vi "Volts_to_temperature_PT__(SubVI).vi"(1 "делитель":dbl, 4 "Resistance":i32, 7 "error in":errorcluster, 16 "Cluster":cluster{"Rref":ext, "Tref":ext, "k":ext}) -> (9 "s? color":u32, 10 "Vin < 0?":bool, 20 "T solvation":dbl, 21 "meas_voltage":dbl, 27 "error out":errorcluster)   [LabVIEW 2015]
uses:
  <vilib>/express/express arith-compare/Formula/XNode/ExpressFormulaBlockNode.xnode
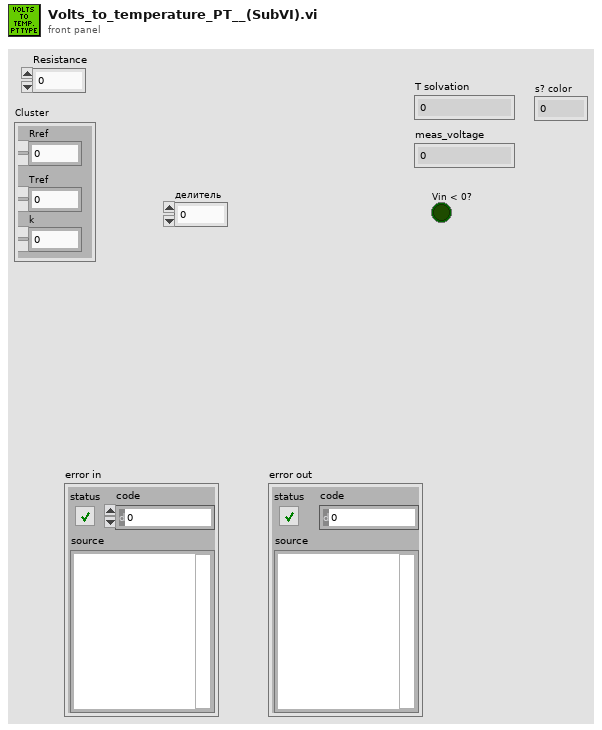
[diagram p1: front panel]
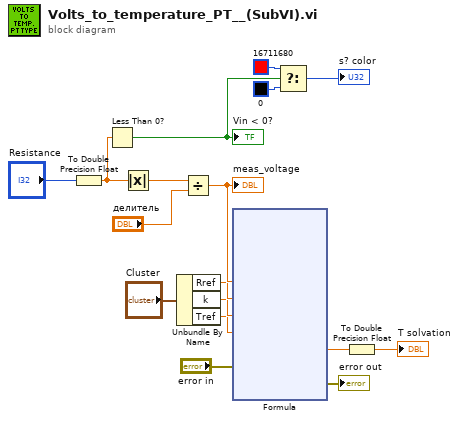
[diagram p0: block diagram]
diagram:
  n1 = To Double Precision Float(number="Resistance") -> (double precision float=w1:dbl)
  n2 = Less Than 0?(x=w1) -> (x < 0?=w15:bool)
  "Vin < 0?" <- w15
  n3 = Absolute Value(x=w1) -> (abs(x)=w13:dbl)
  n4 = Unbundle By Name("Cluster") -> ("Rref"=w5:ext, "k"=w4:ext, "Tref"=w3:ext)
  n5 = Divide(x=w13, y="делитель") -> (x/y=w8:dbl)
  "meas_voltage" <- w8
  n6 = xnode "Formula"("Rt"=w8, "Rref"=w5, "k"=w4, "Tref"=w3, "error in (no error)"="error in") -> ("Result"=w10:ext, "error out"=→"error out":errorcluster)
  n7 = Select(t=u32 16711680, s=w15, f=u32 0) -> (s? t:f=→"s? color":u32)
  n8 = To Double Precision Float(number=w10) -> (double precision float=→"T solvation":dbl)
